vi "Test003-OCR.vi"() -> ()   [LabVIEW 2018]
uses:
  <vilib>/vision/NI_Vision_Development_Module.lvlib
panel:
  in  "X_01":i32=885
  in  "Y_01":i32=300
  in  "W_01":i32=685
  in  "H_01":i32=400
  in  "File Path":path=path "D:/Life/20191001_Accordance/Project/EPISIL/20200806-Camera/LabVIEW_Test/OCR/Train/QQ.bmp"
  in  "TrainFile Path":path=path "D:/Life/20191001_Accordance/Project/EPISIL/20200806-Camera/LabVIEW_Test/OCR"
  out "Show_02 2":T1(plugin-control)
  out "Read String":string
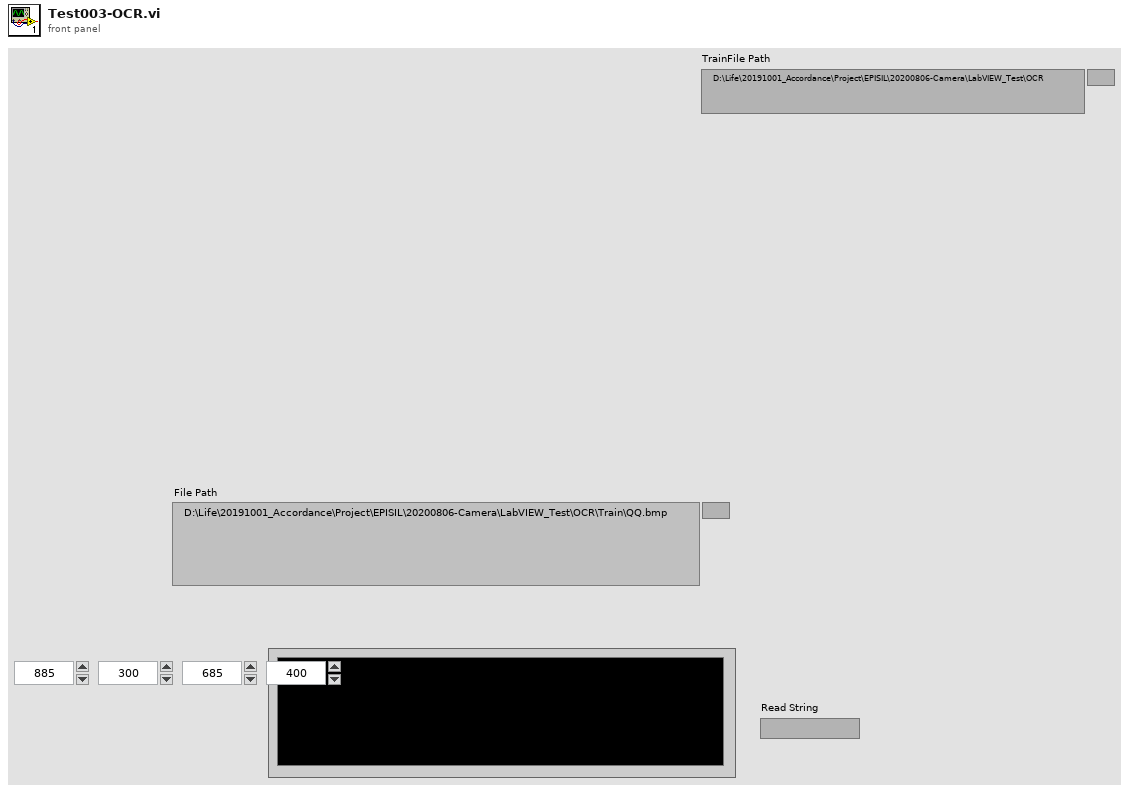
[diagram p1: front panel]
types:
  T1 = typedef "IMAQ Image.ctl" = refnum<image>
  T2 = typedef "IMAQ Rectangle" = cluster{"Left":i32, "Top":i32, "Right":i32, "Bottom":i32, "Rotation":dbl}
  T3 = typedef "Image Type" = u32
  T4 = typedef "ROI Descriptor" = cluster{"Global Rectangle":i32[], "Contours":cluster{"ID":enum32{"External", "Internal"}, "Type":u32, "Coordinates":i32[]}[]}
  T5 = typedef "IMAQ OCR Session.ctl" = refnum<k1>
  T6 = cluster{"Global Rectangle":i32[], "Contours":cluster{"ID":enum32{"External", "Internal"}, "Type":u32, "Coordinates":i32[]}[]}
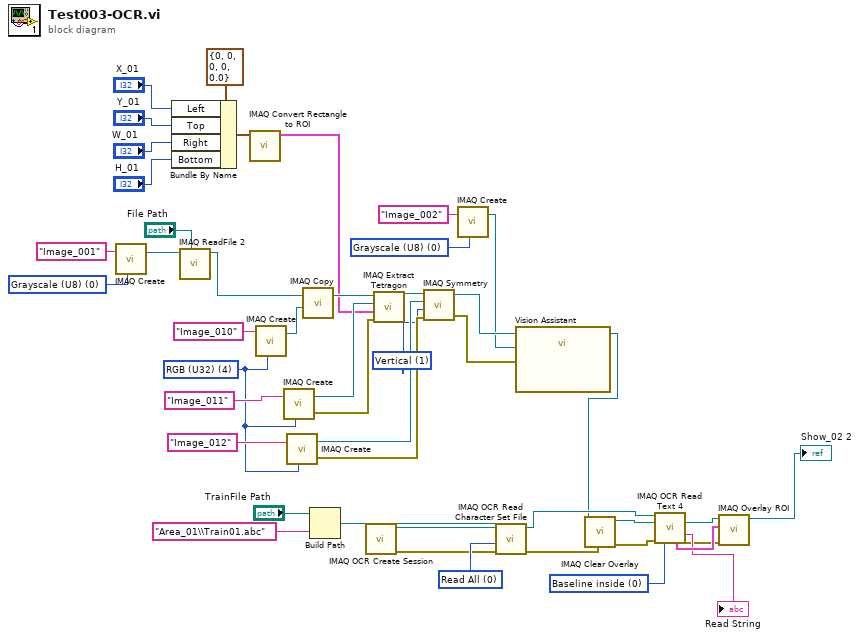
[diagram p0: block diagram]
diagram:
  w14 = u32 1 items=["Horizontal", "Vertical", "Central", "1st Diagonal", "2nd Diagonal"] ("Type of Symmetry")
  w15 = T3 4 items=["Grayscale (U8)", "Grayscale (I16)", "Grayscale (SGL)", "Complex (CSG)", "RGB (U32)", "HSL (U32)", "RGB (U64)", "Grayscale (U16)"] ("Image Type")
  w26 = T3 0 items=["Grayscale (U8)", "Grayscale (I16)", "Grayscale (SGL)", "Complex (CSG)", "RGB (U32)", "HSL (U32)", "RGB (U64)", "Grayscale (U16)"] ("Image Type")
  w27 = u32 0 items=["Baseline inside", "Baseline outside"] ("Orientation")
  w31 = T3 0 items=["Grayscale (U8)", "Grayscale (I16)", "Grayscale (SGL)", "Complex (CSG)", "RGB (U32)", "HSL (U32)", "RGB (U64)", "Grayscale (U16)"] ("Image Type")
  w38 = 0 items=["Read All", "Read Character Set Only", "Read Properties Only"] ("Read Options")
  n1 = call "IMAQ Create"("Image Name"="Image_001", "Image Type"=w31) -> ("New Image"=w29:T1)  [unwired: 3 in, 1 out]
  n2 = Bundle By Name(cluster=T2 {"Left"=0, "Top"=0, "Right"=0, "Bottom"=0, "Rotation"=0.0} ("Rectangle"), "Left"="X_01", "Top"="Y_01", "Right"="W_01", "Bottom"="H_01") -> (w3:T2)
  n3 = call "IMAQ ReadFile 2"("File Path"="File Path", "Image"=w29) -> ("Image Out"=w13:T1)  [unwired: 5 in, 4 out]
  n4 = call "IMAQ Convert Rectangle to ROI"("Rectangle"=w3) -> ("ROI Descriptor"=w1:T4)  [unwired: 8 in, 1 out]
  n5 = call "IMAQ Create"("Image Name"="Image_010", "Image Type"=w15) -> ("New Image"=w18:T1)  [unwired: 3 in, 1 out]
  n6 = call "IMAQ Create"("Image Name"="Image_011", "Image Type"=w15) -> ("New Image"=w20:T1, "error out"=w22:errorcluster)  [unwired: 3 in]
  n7 = call "IMAQ Create"("Image Name"="Image_012", "Image Type"=w15) -> ("New Image"=w21:T1, "error out"=w23:errorcluster)  [unwired: 3 in]
  n8 = call "IMAQ Copy"("Image Dst"=w18, "Image Src"=w13) -> ("Image Dst Out"=w12:T1)  [unwired: 4 in, 1 out]
  n9 = Build Path(base path="TrainFile Path", name or relative path="Area_01\\Train01.abc") -> (appended path=w33:path)
  n10 = call "IMAQ OCR Create Session"() -> ("error out"=w37:errorcluster, "IMAQ OCR Session"=w36:T5)  [unwired: 10 in]
  n11 = call-poly "IMAQ Extract Tetragon"("error in (no error)"=w22, "ROI Descriptor"=w1, "Image Dst"=w20, "Image Src"=w12) -> ("Image Dst Out"=w11:T1)  [unwired: 6 in, 1 out]
  n12 = call "IMAQ Symmetry"("error in (no error)"=w23, "Type of Symmetry"=w14, "Image Dst"=w21, "Image Src"=w11) -> ("error out"=w8:errorcluster, "Image Dst Out"=w10:T1)  [unwired: 1 in]
  n13 = call "IMAQ Create"("Image Name"="Image_002", "Image Type"=w26) -> ("New Image"=w9:T1)  [unwired: 3 in, 1 out]
  n14 = call "IMAQ OCR Read Character Set File"("File Path"=w33, "error in (no error)"=w37, "Read Options"=w38, "IMAQ OCR Session"=w36) -> ("error out"=w41:errorcluster, "IMAQ OCR Session (dup)"=w39:T5)  [unwired: 5 in, 1 out]
  n15 = call "Vision Assistant"("Image In"=w10, "Image Dst"=w9, "error in"=w8) -> ("Image Out"=w25:T1)  [unwired: 23 in, 1 out]
  n16 = call "IMAQ Clear Overlay"("error in (no error)"=w41, "Image"=w25) -> ("error out"=w42:errorcluster, "Image Out"=w40:T1)  [unwired: 8 in]
  n17 = call "IMAQ OCR Read Text 4"("IMAQ OCR Session"=w39, "Image"=w40, "error in (no error)"=w42, "Orientation"=w27) -> ("Image (dup)"=w45:T1, "Read String"=→"Read String":string, "ROI Bounding Characters"=w46:T6, "error out"=w43:errorcluster)  [unwired: 5 in, 3 out]
  n18 = call "IMAQ Overlay ROI"("error in (no error)"=w43, "ROI Descriptor"=w46, "Image"=w45) -> ("Image Out"=→"Show_02 2":T1)  [unwired: 7 in, 1 out]
